vi "SLSCTest Datatype Conversion.vi"() -> (3 "Passed?":bool)   [LabVIEW 2015, in "SLSC EDS Testing.lvlib"]
uses:
  SLSC EDS Testing.lvlib
  <vilib>/Utility/Data Type/Type Definitions/Data Type.ctl
  SLSC UI API/SLSC Tree Control.lvlib
  <vilib>/Utility/Data Type/NI_Data Type.lvlib
panel:
  out "Numeric":i32
  out "U64 2":u64
  out "U64":u64
  out "I32":i32
  out "I8":i8
  out "I64":i64
  out "Reset Variant Check":bool[](array[boolean])
  out "Reset = Value?":bool[](array[boolean])
  out "Value Variant Check":bool[](array[boolean])
  out "String Comparison":bool[](array[boolean])
  out "Value (DBL)":dbl format="%#_16f"
  out "Type":T1
  in  "Ring":u16(ring)
  out "NewVal":variant
  out "Value (DBL)":dbl format="%#_16f"
  out "Value":variant
  out "string data value":string
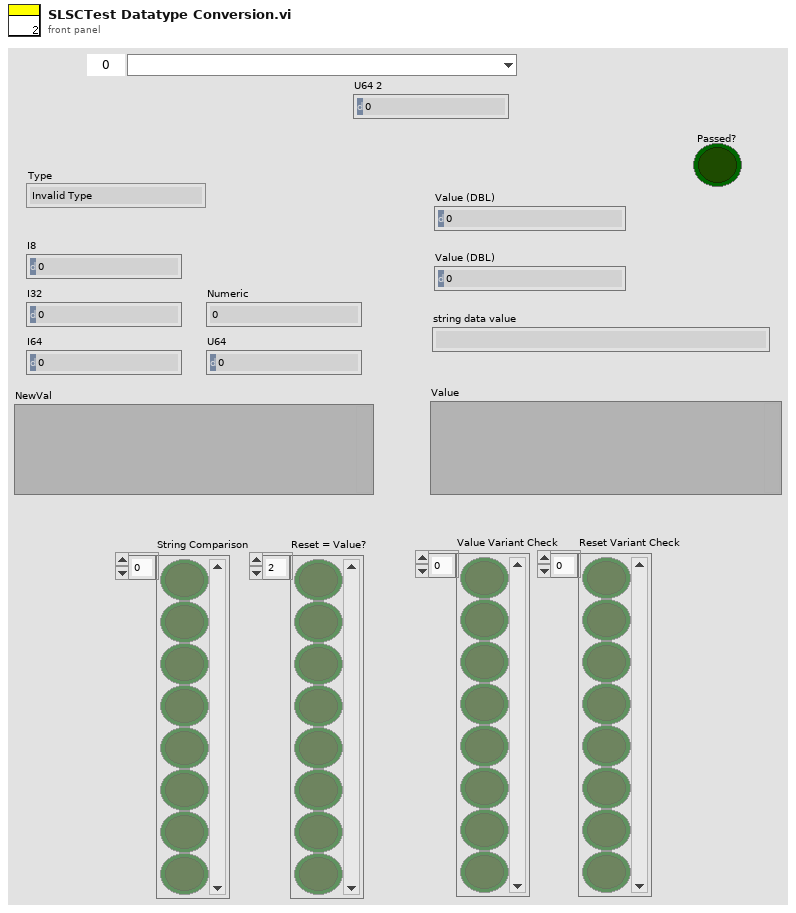
[diagram p1: front panel]
types:
  T1 = typedef "NI_Data Type.lvlib/Data Type.ctl" = enum8{"Invalid Type", "Void", "I8", "I16", "I32", "I64", "U8", "U16", "U32", "U64", "Single Float", "Double Float", "Extended Float", "Single Complex", "Double Complex", "Extended Complex", "Enum U8", "Enum U16", "Enum U32", "Enum U64", "Single Float With Unit", "Double Float With Unit", "Extended Float With Unit", "Single Complex with Unit", "Double Complex with Unit", "Extended Complex with Unit", "Boolean", "String", "Path", "Picture", "Tag", "Array", "Cluster", "Variant", "LV Variant", "Waveform", "Timestamp", "Digital Waveform", "Digital Data", "ExpressData", "Refnum", "External Data", "VI", "Poly VI", "LabVIEW Class Instance", "Fixed Point"}
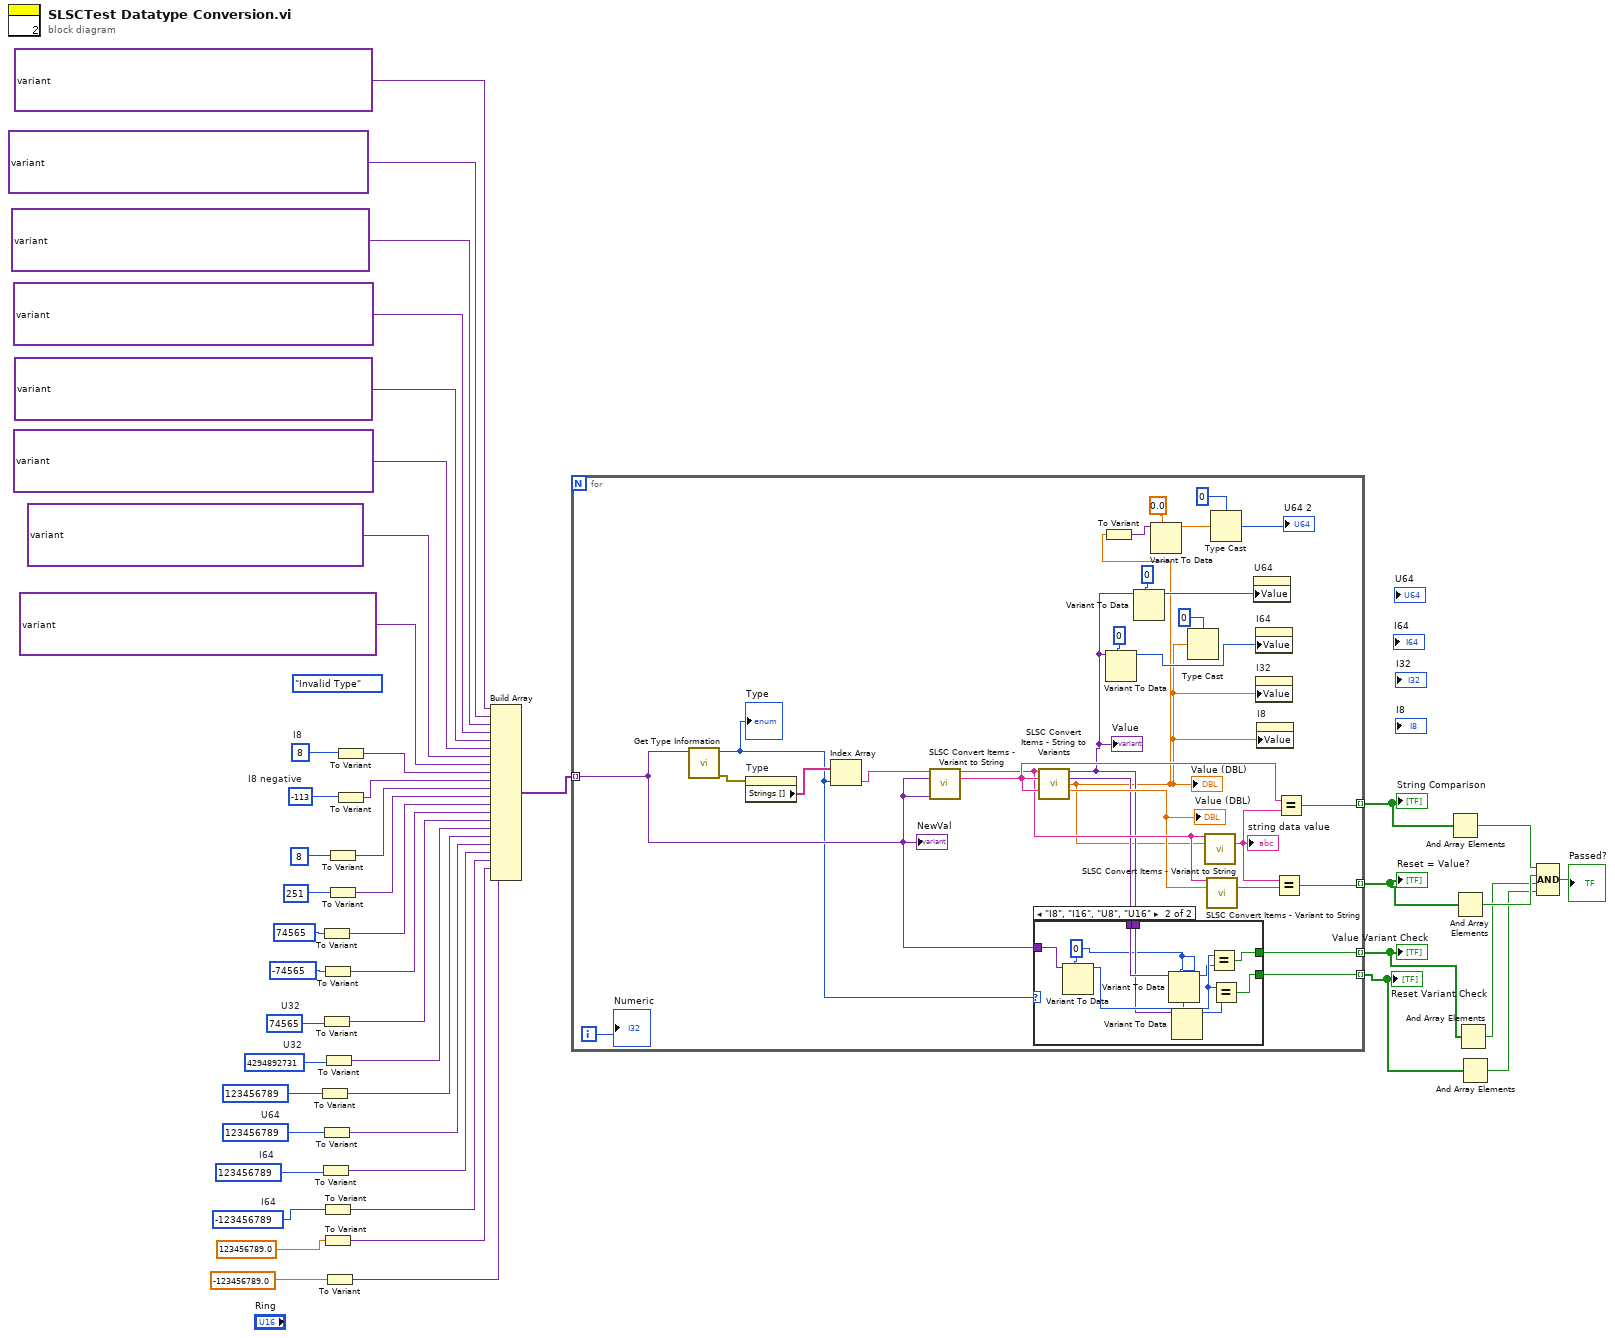
[diagram p0: block diagram]
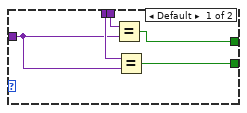
[diagram p2: hidden frame]
diagram:
  w29 = i64 -123456789  # I64
  w31 = u64 123456789  # U64
  w28 = i64 123456789  # I64
  w32 = u32 4294892731  # U32
  w33 = u32 74565  # U32
  (unwired) Data_Type."Invalid Type" ("Type")
  w45 = i8 -113  # I8 negative
  w46 = i8 8  # I8
  n1 = To Variant(anything=u64 123456789 ("U64")) -> (Variant=w25:variant)
  n2 = To Variant(anything=w28) -> (Variant=w23:variant)
  n3 = To Variant(anything=74565 ("I32")) -> (Variant=w36:variant)
  n4 = To Variant(anything=w33) -> (Variant=w27:variant)
  n5 = To Variant(anything=w31) -> (Variant=w24:variant)
  n6 = To Variant(anything=-74565 ("I32")) -> (Variant=w34:variant)
  n7 = To Variant(anything=w29) -> (Variant=w22:variant)
  n8 = To Variant(anything=123456789.0 ("DBL")) -> (Variant=w19:variant)
  n9 = To Variant(anything=w32) -> (Variant=w26:variant)
  n10 = To Variant(anything=-123456789.0 ("DBL")) -> (Variant=w18:variant)
  n11 = To Variant(anything=u8 8 ("U8")) -> (Variant=w40:variant)
  n12 = To Variant(anything=u8 251 ("U8")) -> (Variant=w38:variant)
  n13 = To Variant(anything=w46) -> (Variant=w44:variant)
  n14 = To Variant(anything=w45) -> (Variant=w43:variant)
  n15 = Build Array(variant(i32 -15) ("variant"), variant(u32 241) ("variant"), variant(i32 -3343) ("variant"), variant(u32 62193) ("variant"), variant(i32 -185339151) ("variant"), variant(u32 4109628145) ("variant"), variant(i64 -506664896818842895) ("variant"), variant(u64 17940079176890708721) ("variant"), w44, w43, w40, w38, w36, w34, w27, w26, w25, w24, w23, w22, w19, w18) -> (w42:variant[])
  n16 = for {
    tunnel: w42 -> [w62] mode=indexing
    tunnel: [w66] -> w9 mode=indexing
    tunnel: [w65] -> w8 mode=indexing
    tunnel: [w64] -> w7 mode=indexing
    tunnel: [w61] -> w6 mode=indexing
    i -> [w47]
    n17 = call <vilib>:"Get Type Information.vi"("Variant"=w62) -> ("error out"=w74:errorcluster, "Type"=w55:T1)  [unwired: 6 in, 3 out]
    "Type" <- w55
    n18 = property on="Type" class="Enum (strict)"(error in=w74) -> ("Strings []"=w73:string[])  [unwired: 1 in, 2 out]
    n19 = Index Array(array=w73, index=w55) -> (element=w72:string)
    n20 = call "SLSC Convert Items - Variant to String.vi"("dataType"=w72, "value"=w62, "reset value"=w62) -> ("Output data type"=w70:string, "string data value"=w71:string)  [unwired: 6 in, 5 out]
    n21 = call "SLSC Convert Items - String to Variants.vi"("Datatype"=w70, "Value"=w71, "Reset Value"=w71) -> ("Value"=w52:variant, "Reset Value"=w63:variant, "Value (DBL)"=w49:dbl, "Reset Value (DBL)"=w69:dbl)  [unwired: 9 in]
    "Value (DBL)" <- w49
    "Value" <- w52
    "Value (DBL)" <- w69
    n22 = case shown="\"I8\", \"I16\", \"U8\", \"U16\"" w55 {
      tunnel: [w79 w84] -> w64
      tunnel: w63 -> [w78 w87]
      tunnel: w62 -> [w77 w88]
      tunnel: [w76 w82] -> w61
      tunnel: w52 -> [w75 w83]
      frame Default {
        n23 = Equal?(x=w75, y=w77) -> (x = y?=w79:bool)
        n24 = Equal?(x=w78, y=w77) -> (x = y?=w76:bool)
      }
      frame "I8", "I16", "U8", "U16" {
        w80 = i64 0
        n25 = Variant To Data(type=w80, Variant=w88) -> (data=w86:i64)  [unwired: 1 in, 1 out]
        n26 = Variant To Data(type=w80, Variant=w87) -> (data=w85:i64)  [unwired: 1 in, 1 out]
        n27 = Variant To Data(type=w80, Variant=w83) -> (data=w81:i64)  [unwired: 1 in, 1 out]
        n28 = Equal?(x=w86, y=w85) -> (x = y?=w84:bool)
        n29 = Equal?(x=w86, y=w81) -> (x = y?=w82:bool)
      }
    }
    n30 = To Variant(anything=w49) -> (Variant=w48:variant)
    n31 = Variant To Data(type=i64 0, Variant=w52) -> (data=w58:i64)  [unwired: 1 in, 1 out]
    n32 = Variant To Data(type=u64 0, Variant=w52) -> (data=w56:u64)  [unwired: 1 in, 1 out]
    n33 = Variant To Data(type=0.0, Variant=w48) -> (data=w53:dbl)  [unwired: 1 in, 1 out]
    n34 = Type Cast(type=i64 0 ("I64"), x=w49) -> ()  [unwired: 1 out]
    n35 = call "SLSC Convert Items - Variant to String.vi"("dataType"=w70, "value"=w49) -> ("string data value"=w67:string)  [unwired: 7 in, 6 out]
    "string data value" <- w67
    n36 = call "SLSC Convert Items - Variant to String.vi"("dataType"=w70, "value"=w69) -> ("string data value"=w68:string)  [unwired: 7 in, 6 out]
    n37 = Type Cast(type=i64 0, x=w53) -> (*(type *) &x=→"U64 2":i64)
    n38 = property on="U64" class="DigNum (strict)"("Value"=w56) -> ()  [unwired: 2 in, 2 out]
    n39 = property on="I64" class="DigNum (strict)"("Value"=w58) -> ()  [unwired: 2 in, 2 out]
    n40 = property on="I32" class="DigNum (strict)"("Value"=w49) -> ()  [unwired: 2 in, 2 out]
    n41 = property on="I8" class="DigNum (strict)"("Value"=w49) -> ()  [unwired: 2 in, 2 out]
    n42 = Equal?(x=w67, y=w68) -> (x = y?=w65:bool)
    n43 = Equal?(x=w71, y=w67) -> (x = y?=w66:bool)
    "NewVal" <- w62
    "Numeric" <- w47
  }
  "String Comparison" <- w9
  "Value Variant Check" <- w7
  "Reset = Value?" <- w8
  "Reset Variant Check" <- w6
  n44 = And Array Elements(Boolean array=w9) -> (logical AND=w5:bool)
  n45 = And Array Elements(Boolean array=w8) -> (logical AND=w4:bool)
  n46 = And Array Elements(Boolean array=w7) -> (logical AND=w3:bool)
  n47 = And Array Elements(Boolean array=w6) -> (logical AND=w2:bool)
  n48 = Compound Arithmetic op=AND(w5, w4, w3, w2) -> (→"Passed?":bool)
